vi "restore.vi"(8 "error in (no error)":errorcluster, 11 "plugin in":refnum<class "lv-post-installer.lvclass">) -> (0 "error out":errorcluster, 3 "plugin out":refnum<class "lv-post-installer.lvclass">)   [LabVIEW 2015, in "lv-post-installer.lvlib" / "lv-post-installer.lvclass"]
uses:
  lv-post-installer.lvclass
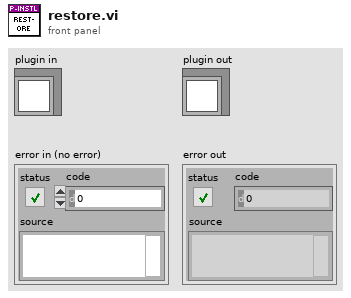
[diagram p1: front panel]
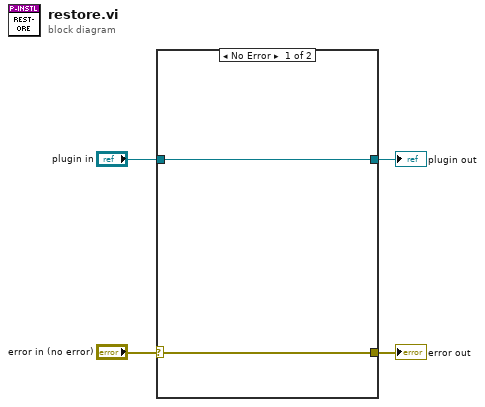
[diagram p0: block diagram]
diagram:
  n1 = case shown="No Error" "error in (no error)" {
    selector: "error in (no error)" -> [w5 w7]
    tunnel: "plugin in" -> [w6 w8]
    tunnel: [w6 w8] -> w3
    tunnel: [w5 w7] -> w1
    frame No Error {
    }
    frame Error {
    }
  }
  "error out" <- w1
  "plugin out" <- w3
